vi "Get Monitor Status.vi"(8 "error in (no error)":errorcluster, 11 "InstrumentHandle_port in":u32) -> (0 "error out":errorcluster, 1 "MonStatus":T1 {"MonStatus" items=["FDX_MON_OFF", "FDX_MON_WAIT_FOR_TRIGGER", "FDX_MON_TRIGGERED", "FDX_MON_STOPPED", "FDX_MON_FULL", "FDX_MON_OVERLOAD"]}, 3 "InstrumentHandle_port out":u32)   [LabVIEW 2020, in "AIM664LV.lvlib"]
uses:
  AIM664LV.lvlib
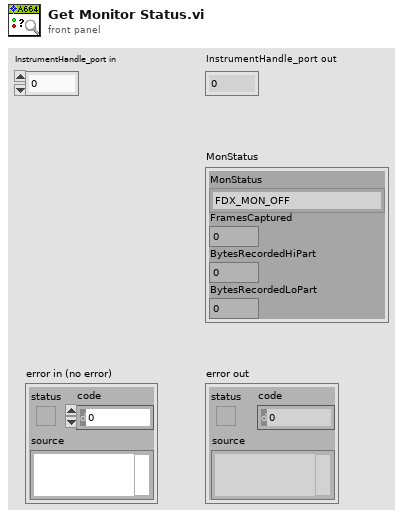
[diagram p1: front panel]
types:
  T1 = cluster{"MonStatus":u32, "FramesCaptured":u32, "BytesRecordedHiPart":u32, "BytesRecordedLoPart":u32}
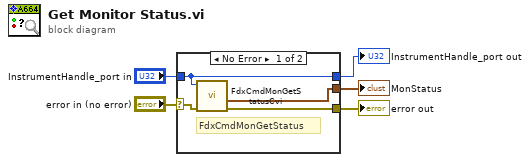
[diagram p0: block diagram]
diagram:
  n1 = case shown="No Error" "error in (no error)" {
    selector: "error in (no error)" -> [w8 w10]
    tunnel: "InstrumentHandle_port in" -> [w9 w11]
    tunnel: [w7 w10] -> w3
    tunnel: [w9 w11] -> w2
    tunnel: [w6 _] -> w1
    frame No Error {
      # "FdxCmdMonGetStatus"
      n2 = call "FdxCmdMonGetStatusCvi.vi"("error in"=w8, "InstrumentHandle_port"=w9) -> ("error out"=w7:errorcluster, "MonStatus"=w6:T1)  [unwired: 7 in, 1 out]
    }
    frame Error {
    }
  }
  "error out" <- w3
  "InstrumentHandle_port out" <- w2
  "MonStatus" <- w1
